vi "1.vi"(0 "输入":dbl) -> (1 "余弦":dbl, 2 "正弦":dbl)   [LabVIEW 2017]
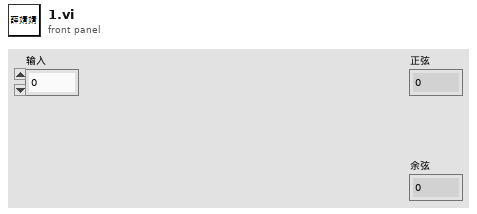
[diagram p1: front panel]
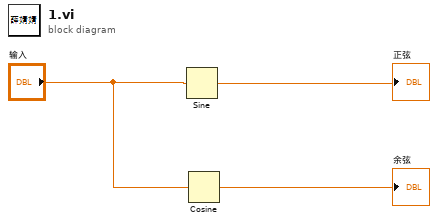
[diagram p0: block diagram]
diagram:
  n1 = Sine(x="输入") -> (sin(x)=→"正弦":dbl)
  n2 = Cosine(x="输入") -> (cos(x)=→"余弦":dbl)
